vi "GDFgetWaveformArrayRefnum.vi"(8 "error in (no error)":errorcluster, 11 "GDFv1.x in":refnum<class "GDFv1.x.lvclass">) -> (0 "error out":errorcluster, 2 "GDFv1.x out":refnum<class "GDFv1.x.lvclass">, 3 "Waveform array reference":refnum<data-value>)   [LabVIEW 2016, in "GDF File Reader.lvlib" / "GDFv1.x.lvclass"]
uses:
  GDFv1.x.lvclass
  GDFv1.x.lvclass/GDFv1.x.ctl
panel:
  # "This VI is a part of BCI Design library, http://www.ru-bci.org \nCopyright © 2020, Sotnikov Peter, All rights reserved. License: GNU GPLv3"
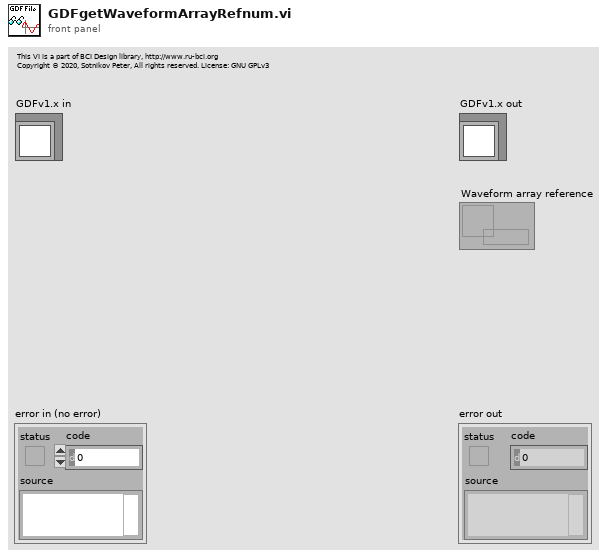
[diagram p1: front panel]
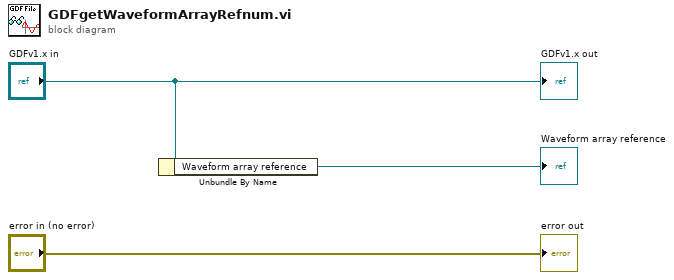
[diagram p0: block diagram]
diagram:
  n1 = Unbundle By Name("GDFv1.x in") -> ("Waveform array reference"=→"Waveform array reference":refnum<data-value>)
  "error out" <- "error in (no error)"
  "GDFv1.x out" <- "GDFv1.x in"
